vi "Lossy Enqueue Message (Array).vi"(6 "Priority Message? Array":bool[](array[boolean]), 8 "error in (no error)":errorcluster, 9 "Message Data Array":variant[](array[variant]), 10 "Message Array":string[](array[string]), 11 "Message Queue":refnum<queue>) -> (0 "error out":errorcluster, 3 "dup Message Queue":refnum<queue>)   [LabVIEW 2014, in "Message Queue.lvlib"]
doc: "For a regular message, enqueue the message. For a priority message, enqueue it at the front of the queue."
uses:
  Message Queue.lvlib
  Message Cluster.ctl
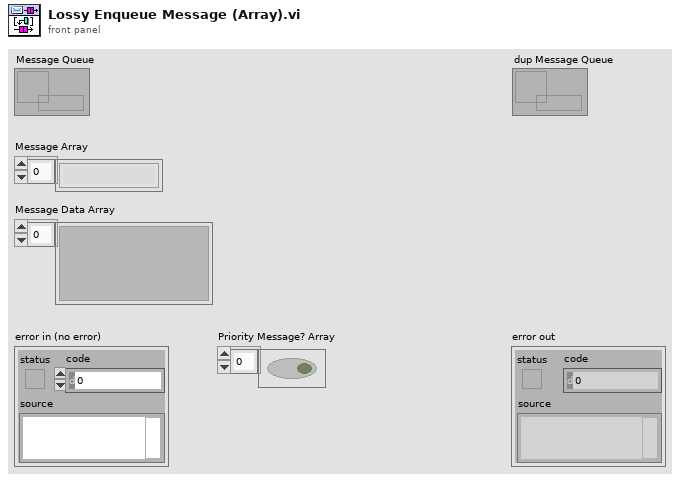
[diagram p1: front panel]
types:
  T1 = typedef "Message Queue.lvlib/Message Cluster.ctl" = cluster{"Message":string, "Message Data":variant}
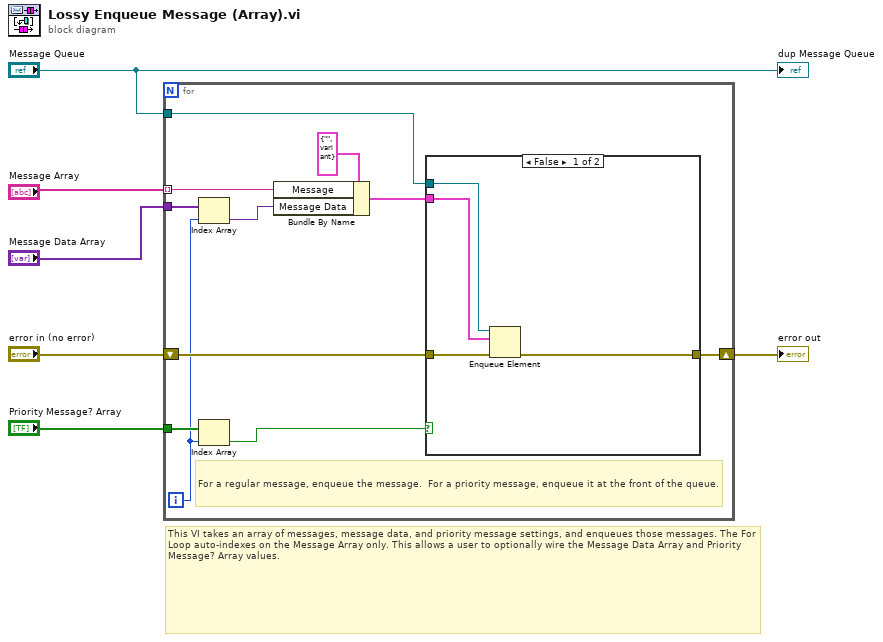
[diagram p0: block diagram]
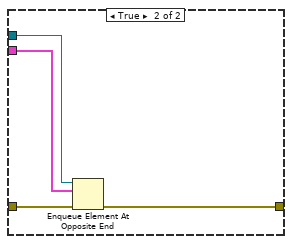
[diagram p2: hidden frame]
diagram:
  # "This VI takes an array of messages, message data, and priority message settings, and enqueues those messages. The For Loop auto-indexes on the Message Array only. This allows a user to optionally wire the Message Data Array and Priority Message? Array values."
  n1 = for {
    tunnel: "Message Array" -> [w16] mode=indexing
    tunnel: "Message Data Array" -> [w11]
    tunnel: "Priority Message? Array" -> [w9]
    tunnel: "Message Queue" -> [w13]
    shift-right: [w14] -> w2
    shift-left: "error in (no error)" -> [w15]
    i -> [w7]
    # "For a regular message, enqueue the message.  For a priority message, enqueue it at the front of the queue."
    n2 = Index Array(array=w11, index=w7) -> (element=w10:variant)
    n3 = Index Array(array=w9, index=w7) -> (element=w8:bool)
    n4 = Bundle By Name(cluster=T1 {"Message"="", "Message Data"=variant} ("Message Cluster"), "Message"=w16, "Message Data"=w10) -> (w12:T1)
    n5 = case shown="False" w8 {
      tunnel: w15 -> [w21 w25]
      tunnel: [w20 w24] -> w14
      tunnel: w13 -> [w19 w23]
      tunnel: w12 -> [w18 w22]
      frame False {
        n6 = Enqueue Element(queue=w19, element=w18, error in (no error)=w21) -> (error out=w20:errorcluster)  [unwired: 1 in, 2 out]
      }
      frame True {
        n7 = Enqueue Element At Opposite End(queue=w23, element=w22, error in (no error)=w25) -> (error out=w24:errorcluster)  [unwired: 1 in, 2 out]
      }
    }
  }
  "error out" <- w2
  "dup Message Queue" <- "Message Queue"
